vi "PCO_GetAcqEnblSignalStatus.vi"(8 "error in (no error)":errorcluster {"code" format="%x"}, 11 "ph":u64) -> (0 "error out":errorcluster {"code" format="%x"}, 1 "wAcquEnableState":u16(ring) items=["FALSE", "TRUE"], 2 "ErrorMessage":i32 format="%x", 3 "ph out":u64)   [LabVIEW 2019, in "SDK.lvlib" / "RecordingControl.lvlib"]
doc: "<b>Description:</b>\nThis function returns the current status of the external <acq enbl> input. Depending on the I/O configuration a high or low level at the external <acq enbl> input does set the acquire enable state to TRUE.\nDue to response and processing times the delay between the delivered status and the current status may be several 10 ms e.g. caused by the interface and/or the operating system.\nIf timing is critical it is strongly recommended to use other trigger modes.\n\n<b>Supported camera type:</b>\npco.1600, pco.2000, pco.4000\n\n<b>Descriptor dependency:</b>\ndwGeneralCapsDESC1: NO_ACQUIREMODE"
uses:
  RecordingControl.lvlib
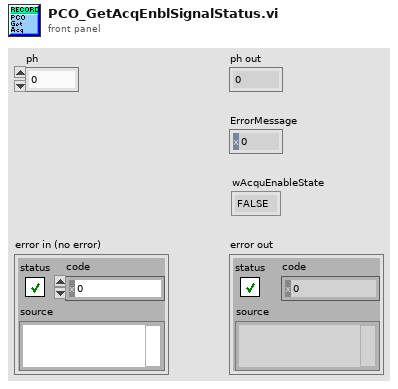
[diagram p1: front panel]
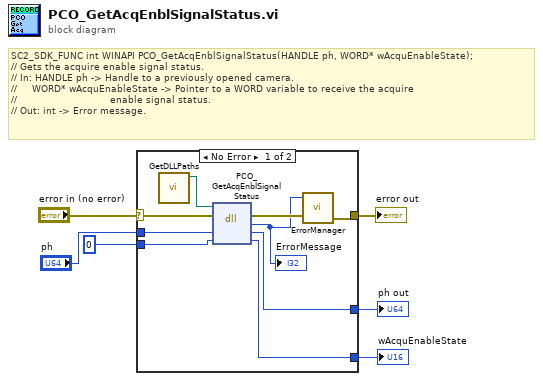
[diagram p0: block diagram]
diagram:
  # "SC2_SDK_FUNC int WINAPI PCO_GetAcqEnblSignalStatus(HANDLE ph, WORD* wAcquEnableState);\n// Gets the acquire enable signal status.\n// In: HANDLE ph -> Handle to a previously opened camera.\n//     WORD* wAcquEnableState -> Pointer to a WORD variable to receive the acquire\n//                               enable signal status.\n// Out: int -> Error message."
  n1 = case shown="No Error" "error in (no error)" {
    selector: "error in (no error)" -> [w11 w18]
    tunnel: "ph" -> [w15 w17]
    tunnel: [w14 w17] -> w5
    tunnel: u16 0 ("wAcquEnableState") -> [w13 w16]
    tunnel: [w12 w16] -> w3
    tunnel: [w9 w18] -> w2
    frame No Error {
      n2 = call "GetDLLPaths.vi"() -> ("SC2_Cam_Path"=w7:path)  [unwired: 9 in, 2 out]
      n3 = dll-call lib="?" fn="PCO_GetAcqEnblSignalStatus"(path in=w7, error in=w11, "ph"=w15, "wAcquEnableState"=w13) -> (error out=w10:errorcluster, "return type"=w8:i32, "ph"=w14:u64, "wAcquEnableState"=w12:u16)  [unwired: 1 in, 1 out]
      "ErrorMessage" <- w8
      n4 = call "ErrorManager.vi"("error in (no error)"=w10, "error code"=w8) -> ("error out"=w9:errorcluster)  [unwired: 3 in]
    }
    frame Error {
    }
  }
  "ph out" <- w5
  "wAcquEnableState" <- w3
  "error out" <- w2
